vi "subvi Robot Get Motor Position.vi"(0 "VISA In":refnum<visa-resource-name>, 1 "Motor Number":i32=1 min=1 max=4 step=1) -> (2 "Success":bool, 3 "VISA Out":refnum<visa-resource-name>, 4 "Motor Position":string, 5 "error out":errorcluster)   [LabVIEW 2012]
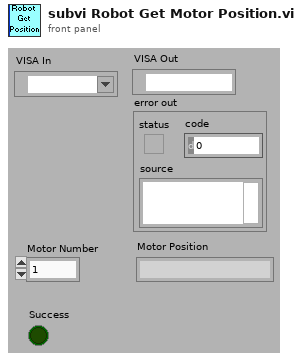
[diagram p1: front panel]
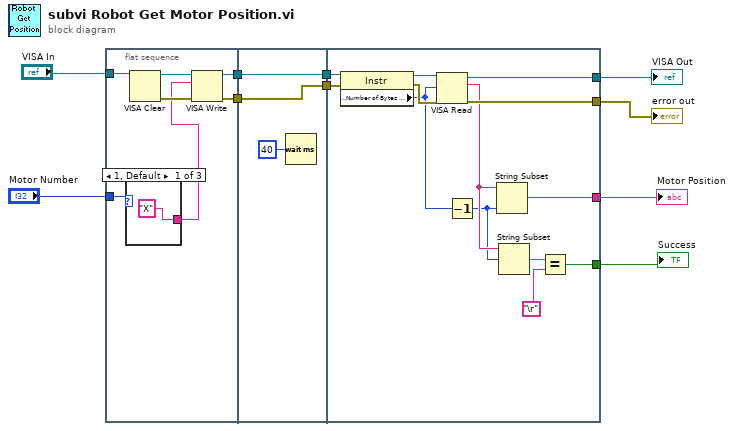
[diagram p0: block diagram]
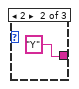
[diagram p2: hidden frame]
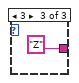
[diagram p3: hidden frame]
diagram:
  n1 = flat-sequence {
    tunnel: "Motor Number" -> [w12]
    tunnel: "VISA In" -> [w17]
    tunnel: [w14] -> w9
    tunnel: [w13] -> w7
    tunnel: [w22] -> w10
    tunnel: w9 -> [w22]
    tunnel: [w21] -> w8
    tunnel: w7 -> [w21]
    tunnel: w10 -> [w36]
    tunnel: w8 -> [w35]
    tunnel: [w32] -> w2
    tunnel: [w31] -> w3
    tunnel: [w29] -> w6
    tunnel: [w24] -> w4
    frame #0 {
      n2 = case shown="1, Default" w12 {
        tunnel: ["X" ("write buffer") "Y" "Z"] -> w11
        frame 1, Default {
        }
        frame 2 {
        }
        frame 3 {
        }
      }
      n3 = VISA Clear(VISA resource name=w17) -> (VISA resource name out=w16:refnum<visa-resource-name>, error out=w15:errorcluster)  [unwired: 1 in]
      n4 = VISA Write(VISA resource name=w16, write buffer=w11, error in (no error)=w15) -> (VISA resource name out=w14:refnum<visa-resource-name>, error out=w13:errorcluster)  [unwired: 1 out]
    }
    frame #1 {
      n5 = Wait (ms)(milliseconds to wait=u32 40) -> ()  [unwired: 1 out]
    }
    frame #2 {
      n6 = property class="Instr"(reference=w36, error in=w35) -> (reference out=w34:refnum<visa-resource-name>, error out=w33:errorcluster, "Serial Settings:Number of Bytes at Serial Port"=w30:u32)
      n7 = VISA Read(VISA resource name=w34, byte count=w30, error in (no error)=w33) -> (VISA resource name out=w32:refnum<visa-resource-name>, read buffer=w28:string, error out=w31:errorcluster)  [unwired: 1 out]
      n8 = Decrement(x=w30) -> (x-1=w27:u32)
      n9 = String Subset(string=w28, length (rest)=w27) -> (substring=w29:string)  [unwired: 1 out]
      n10 = String Subset(string=w28, offset (0)=w27) -> (substring=w26:string)  [unwired: 1 out]
      n11 = Equal?(x=w26, y="\r") -> (x = y?=w24:bool)
    }
  }
  "VISA Out" <- w2
  "error out" <- w3
  "Motor Position" <- w6
  "Success" <- w4
